vi "ArmSetChickenEnable.vi"(8 "ChickenEnable":bool) -> ()   [LabVIEW 2020]
doc: "Setter for ArmChickenEnable\nInputs:\n--ChickenEnable--Boolean--"
uses:
  ArmGlobal.vi
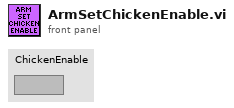
[diagram p1: front panel]
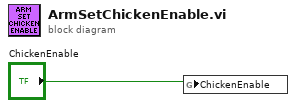
[diagram p0: block diagram]
diagram:
  n1 = global write "ArmGlobal.vi" "ChickenEnable"("ChickenEnable") -> ()
